vi "String to Boolean Array.vi"(8 "error in (no error)":errorcluster, 11 "String":string) -> (0 "error out":errorcluster, 2 "Array":bool[][](array[boolean]))   [LabVIEW 2026, in "LED Matrix.lvlib" / "Text.lvclass"]
uses:
  Text.lvclass
  Text.lvclass/Text.ctl
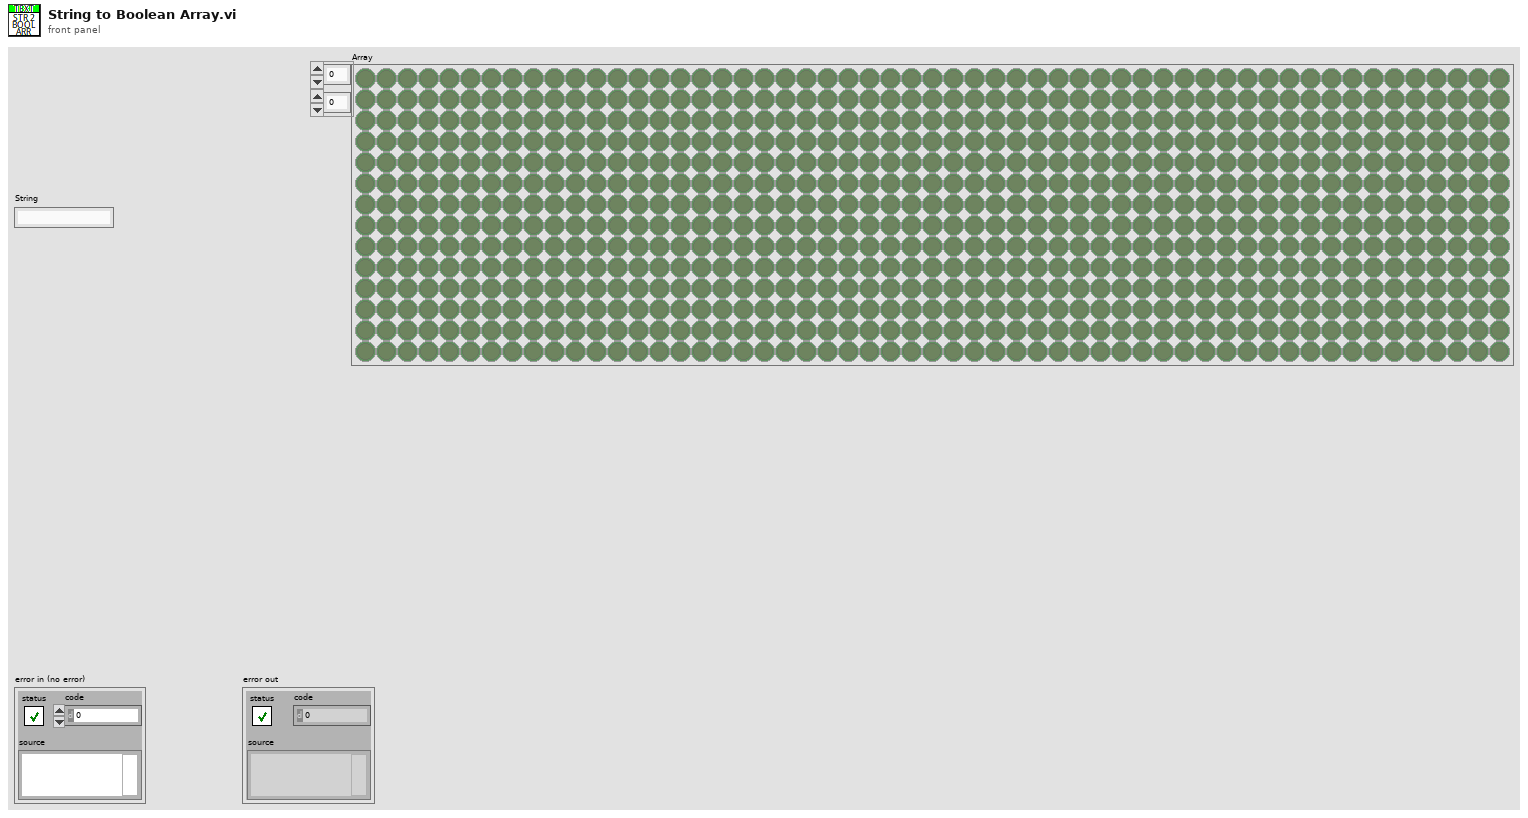
[diagram p1: front panel]
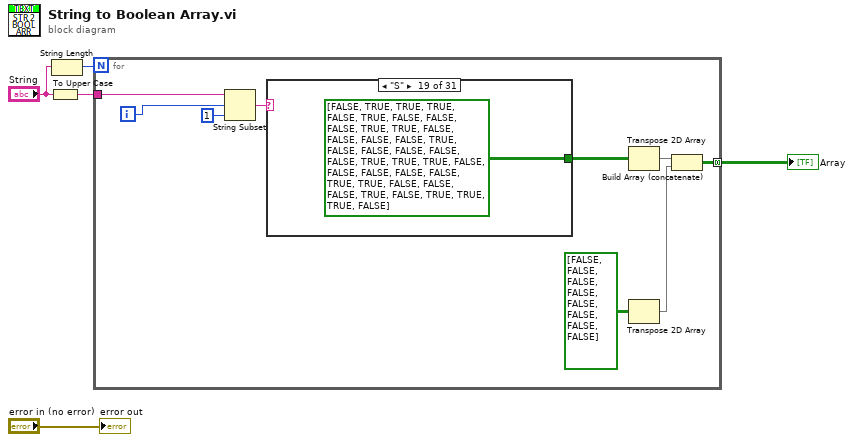
[diagram p0: block diagram]
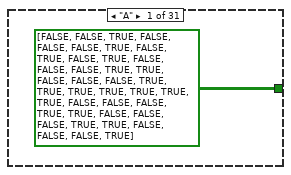
[diagram p2: hidden frame]
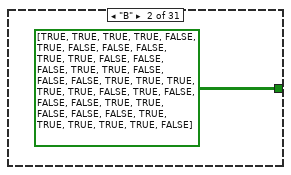
[diagram p3: hidden frame]
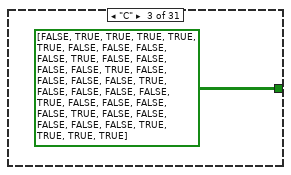
[diagram p4: hidden frame]
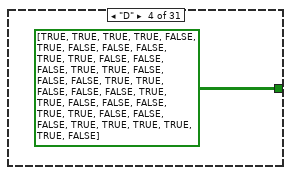
[diagram p5: hidden frame]
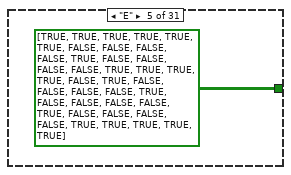
[diagram p6: hidden frame]
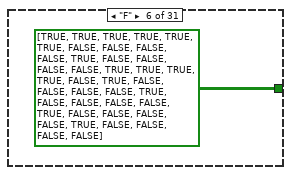
[diagram p7: hidden frame]
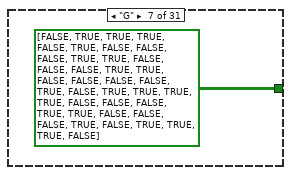
[diagram p8: hidden frame]
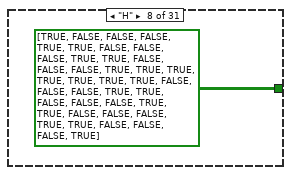
[diagram p9: hidden frame]
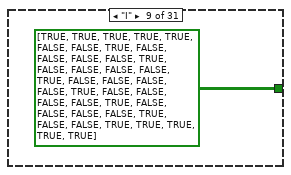
[diagram p10: hidden frame]
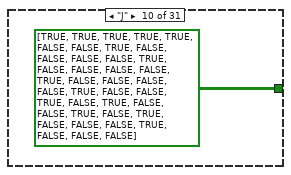
[diagram p11: hidden frame]
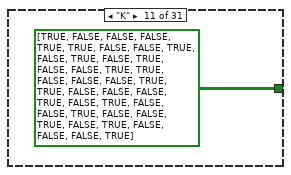
[diagram p12: hidden frame]
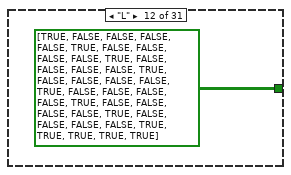
[diagram p13: hidden frame]
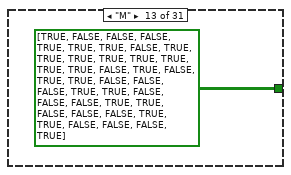
[diagram p14: hidden frame]
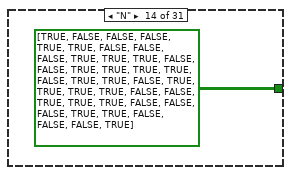
[diagram p15: hidden frame]
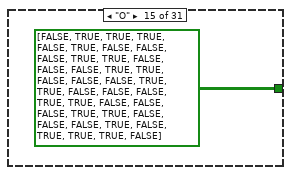
[diagram p16: hidden frame]
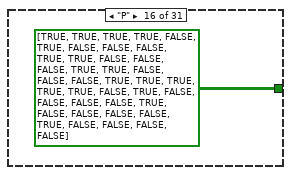
[diagram p17: hidden frame]
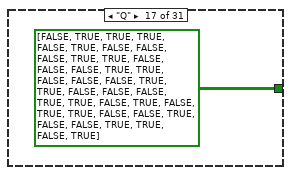
[diagram p18: hidden frame]
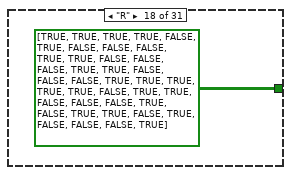
[diagram p19: hidden frame]
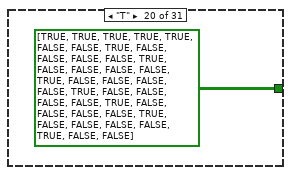
[diagram p20: hidden frame]
diagram:
  n1 = To Upper Case(1:"String") -> (0:w1:string)
  n2 = String Length(string="String") -> (length=w5:i32)
  n3 = for {
    N: w5 -> [_]
    tunnel: w1 -> [w14]
    tunnel: [w8] -> w3 mode=concatenating
    i -> [w9]
    n4 = String Subset(string=w14, offset (0)=w9, length (rest)=1 ("length (rest)")) -> (substring=w12:string)
    n5 = case shown="\"S\"" w12 {
      tunnel: [bool[][] [[FALSE, FALSE, TRUE, FALSE, FALSE], [FALSE, TRUE, FALSE, TRUE, FALSE], [TRUE, FALSE, FALSE, FALSE, TRUE], [TRUE, FALSE, FALSE, FALSE, TRUE], [TRUE, TRUE, TRUE, TRUE, TRUE], [TRUE, FALSE, FALSE, FALSE, TRUE], [TRUE, FALSE, FALSE, FALSE, TRUE], [TRUE, FALSE, FALSE, FALSE, TRUE]] bool[][] [[TRUE, TRUE, TRUE, TRUE, FALSE], [TRUE, FALSE, FALSE, FALSE, TRUE], [TRUE, FALSE, FALSE, FALSE, TRUE], [TRUE, FALSE, FALSE, FALSE, TRUE], [TRUE, TRUE, TRUE, TRUE, FALSE], [TRUE, FALSE, FALSE, FALSE, TRUE], [TRUE, FALSE, FALSE, FALSE, TRUE], [TRUE, TRUE, TRUE, TRUE, FALSE]] bool[][] [[FALSE, TRUE, TRUE, TRUE, TRUE], [TRUE, FALSE, FALSE, FALSE, FALSE], [TRUE, FALSE, FALSE, FALSE, FALSE], [TRUE, FALSE, FALSE, FALSE, FALSE], [TRUE, FALSE, FALSE, FALSE, FALSE], [TRUE, FALSE, FALSE, FALSE, FALSE], [TRUE, FALSE, FALSE, FALSE, FALSE], [FALSE, TRUE, TRUE, TRUE, TRUE]] bool[][] [[TRUE, TRUE, TRUE, TRUE, FALSE], [TRUE, FALSE, FALSE, FALSE, TRUE], [TRUE, FALSE, FALSE, FALSE, TRUE], [TRUE, FALSE, FALSE, FALSE, TRUE], [TRUE, FALSE, FALSE, FALSE, TRUE], [TRUE, FALSE, FALSE, FALSE, TRUE], [TRUE, FALSE, FALSE, FALSE, TRUE], [TRUE, TRUE, TRUE, TRUE, FALSE]] bool[][] [[TRUE, TRUE, TRUE, TRUE, TRUE], [TRUE, FALSE, FALSE, FALSE, FALSE], [TRUE, FALSE, FALSE, FALSE, FALSE], [TRUE, TRUE, TRUE, TRUE, FALSE], [TRUE, FALSE, FALSE, FALSE, FALSE], [TRUE, FALSE, FALSE, FALSE, FALSE], [TRUE, FALSE, FALSE, FALSE, FALSE], [TRUE, TRUE, TRUE, TRUE, TRUE]] bool[][] [[TRUE, TRUE, TRUE, TRUE, TRUE], [TRUE, FALSE, FALSE, FALSE, FALSE], [TRUE, FALSE, FALSE, FALSE, FALSE], [TRUE, TRUE, TRUE, TRUE, FALSE], [TRUE, FALSE, FALSE, FALSE, FALSE], [TRUE, FALSE, FALSE, FALSE, FALSE], [TRUE, FALSE, FALSE, FALSE, FALSE], [TRUE, FALSE, FALSE, FALSE, FALSE]] bool[][] [[FALSE, TRUE, TRUE, TRUE, FALSE], [TRUE, FALSE, FALSE, FALSE, TRUE], [TRUE, FALSE, FALSE, FALSE, TRUE], [TRUE, FALSE, FALSE, FALSE, FALSE], [TRUE, FALSE, TRUE, TRUE, TRUE], [TRUE, FALSE, FALSE, FALSE, TRUE], [TRUE, FALSE, FALSE, FALSE, TRUE], [FALSE, TRUE, TRUE, TRUE, FALSE]] bool[][] [[TRUE, FALSE, FALSE, FALSE, TRUE], [TRUE, FALSE, FALSE, FALSE, TRUE], [TRUE, FALSE, FALSE, FALSE, TRUE], [TRUE, TRUE, TRUE, TRUE, TRUE], [TRUE, FALSE, FALSE, FALSE, TRUE], [TRUE, FALSE, FALSE, FALSE, TRUE], [TRUE, FALSE, FALSE, FALSE, TRUE], [TRUE, FALSE, FALSE, FALSE, TRUE]] bool[][] [[TRUE, TRUE, TRUE, TRUE, TRUE], [FALSE, FALSE, TRUE, FALSE, FALSE], [FALSE, FALSE, TRUE, FALSE, FALSE], [FALSE, FALSE, TRUE, FALSE, FALSE], [FALSE, FALSE, TRUE, FALSE, FALSE], [FALSE, FALSE, TRUE, FALSE, FALSE], [FALSE, FALSE, TRUE, FALSE, FALSE], [TRUE, TRUE, TRUE, TRUE, TRUE]] bool[][] [[TRUE, TRUE, TRUE, TRUE, TRUE], [FALSE, FALSE, TRUE, FALSE, FALSE], [FALSE, FALSE, TRUE, FALSE, FALSE], [FALSE, FALSE, TRUE, FALSE, FALSE], [FALSE, FALSE, TRUE, FALSE, FALSE], [TRUE, FALSE, TRUE, FALSE, FALSE], [TRUE, FALSE, TRUE, FALSE, FALSE], [FALSE, TRUE, FALSE, FALSE, FALSE]] bool[][] [[TRUE, FALSE, FALSE, FALSE, TRUE], [TRUE, FALSE, FALSE, TRUE, FALSE], [TRUE, FALSE, TRUE, FALSE, FALSE], [TRUE, TRUE, FALSE, FALSE, FALSE], [TRUE, TRUE, FALSE, FALSE, FALSE], [TRUE, FALSE, TRUE, FALSE, FALSE], [TRUE, FALSE, FALSE, TRUE, FALSE], [TRUE, FALSE, FALSE, FALSE, TRUE]] bool[][] [[TRUE, FALSE, FALSE, FALSE, FALSE], [TRUE, FALSE, FALSE, FALSE, FALSE], [TRUE, FALSE, FALSE, FALSE, FALSE], [TRUE, FALSE, FALSE, FALSE, FALSE], [TRUE, FALSE, FALSE, FALSE, FALSE], [TRUE, FALSE, FALSE, FALSE, FALSE], [TRUE, FALSE, FALSE, FALSE, FALSE], [TRUE, TRUE, TRUE, TRUE, TRUE]] bool[][] [[TRUE, FALSE, FALSE, FALSE, TRUE], [TRUE, TRUE, FALSE, TRUE, TRUE], [TRUE, TRUE, TRUE, TRUE, TRUE], [TRUE, FALSE, TRUE, FALSE, TRUE], [TRUE, FALSE, FALSE, FALSE, TRUE], [TRUE, FALSE, FALSE, FALSE, TRUE], [TRUE, FALSE, FALSE, FALSE, TRUE], [TRUE, FALSE, FALSE, FALSE, TRUE]] bool[][] [[TRUE, FALSE, FALSE, FALSE, TRUE], [TRUE, FALSE, FALSE, FALSE, TRUE], [TRUE, TRUE, FALSE, FALSE, TRUE], [TRUE, TRUE, TRUE, FALSE, TRUE], [TRUE, FALSE, TRUE, TRUE, TRUE], [TRUE, FALSE, FALSE, TRUE, TRUE], [TRUE, FALSE, FALSE, FALSE, TRUE], [TRUE, FALSE, FALSE, FALSE, TRUE]] bool[][] [[FALSE, TRUE, TRUE, TRUE, FALSE], [TRUE, FALSE, FALSE, FALSE, TRUE], [TRUE, FALSE, FALSE, FALSE, TRUE], [TRUE, FALSE, FALSE, FALSE, TRUE], [TRUE, FALSE, FALSE, FALSE, TRUE], [TRUE, FALSE, FALSE, FALSE, TRUE], [TRUE, FALSE, FALSE, FALSE, TRUE], [FALSE, TRUE, TRUE, TRUE, FALSE]] bool[][] [[TRUE, TRUE, TRUE, TRUE, FALSE], [TRUE, FALSE, FALSE, FALSE, TRUE], [TRUE, FALSE, FALSE, FALSE, TRUE], [TRUE, FALSE, FALSE, FALSE, TRUE], [TRUE, TRUE, TRUE, TRUE, FALSE], [TRUE, FALSE, FALSE, FALSE, FALSE], [TRUE, FALSE, FALSE, FALSE, FALSE], [TRUE, FALSE, FALSE, FALSE, FALSE]] bool[][] [[FALSE, TRUE, TRUE, TRUE, FALSE], [TRUE, FALSE, FALSE, FALSE, TRUE], [TRUE, FALSE, FALSE, FALSE, TRUE], [TRUE, FALSE, FALSE, FALSE, TRUE], [TRUE, FALSE, FALSE, FALSE, TRUE], [TRUE, FALSE, TRUE, FALSE, TRUE], [TRUE, FALSE, FALSE, TRUE, FALSE], [FALSE, TRUE, TRUE, FALSE, TRUE]] bool[][] [[TRUE, TRUE, TRUE, TRUE, FALSE], [TRUE, FALSE, FALSE, FALSE, TRUE], [TRUE, FALSE, FALSE, FALSE, TRUE], [TRUE, FALSE, FALSE, FALSE, TRUE], [TRUE, TRUE, TRUE, TRUE, FALSE], [TRUE, TRUE, FALSE, FALSE, FALSE], [TRUE, FALSE, TRUE, TRUE, FALSE], [TRUE, FALSE, FALSE, FALSE, TRUE]] bool[][] [[FALSE, TRUE, TRUE, TRUE, FALSE], [TRUE, FALSE, FALSE, FALSE, TRUE], [TRUE, FALSE, FALSE, FALSE, FALSE], [TRUE, FALSE, FALSE, FALSE, FALSE], [FALSE, TRUE, TRUE, TRUE, FALSE], [FALSE, FALSE, FALSE, FALSE, TRUE], [TRUE, FALSE, FALSE, FALSE, TRUE], [FALSE, TRUE, TRUE, TRUE, FALSE]] bool[][] [[TRUE, TRUE, TRUE, TRUE, TRUE], [FALSE, FALSE, TRUE, FALSE, FALSE], [FALSE, FALSE, TRUE, FALSE, FALSE], [FALSE, FALSE, TRUE, FALSE, FALSE], [FALSE, FALSE, TRUE, FALSE, FALSE], [FALSE, FALSE, TRUE, FALSE, FALSE], [FALSE, FALSE, TRUE, FALSE, FALSE], [FALSE, FALSE, TRUE, FALSE, FALSE]] bool[][] [[TRUE, FALSE, FALSE, FALSE, TRUE], [TRUE, FALSE, FALSE, FALSE, TRUE], [TRUE, FALSE, FALSE, FALSE, TRUE], [TRUE, FALSE, FALSE, FALSE, TRUE], [TRUE, FALSE, FALSE, FALSE, TRUE], [TRUE, FALSE, FALSE, FALSE, TRUE], [TRUE, FALSE, FALSE, FALSE, TRUE], [FALSE, TRUE, TRUE, TRUE, FALSE]] bool[][] [[TRUE, FALSE, FALSE, FALSE, TRUE], [TRUE, FALSE, FALSE, FALSE, TRUE], [TRUE, FALSE, FALSE, FALSE, TRUE], [TRUE, FALSE, FALSE, FALSE, TRUE], [FALSE, TRUE, FALSE, TRUE, FALSE], [FALSE, TRUE, FALSE, TRUE, FALSE], [FALSE, TRUE, FALSE, TRUE, FALSE], [FALSE, FALSE, TRUE, FALSE, FALSE]] bool[][] [[TRUE, FALSE, FALSE, FALSE, FALSE, FALSE, FALSE, FALSE, TRUE], [TRUE, FALSE, FALSE, FALSE, FALSE, FALSE, FALSE, FALSE, TRUE], [TRUE, FALSE, FALSE, FALSE, FALSE, FALSE, FALSE, FALSE, TRUE], [TRUE, FALSE, FALSE, FALSE, TRUE, FALSE, FALSE, FALSE, TRUE], [FALSE, TRUE, FALSE, TRUE, FALSE, TRUE, FALSE, TRUE, FALSE], [FALSE, TRUE, FALSE, TRUE, FALSE, TRUE, FALSE, TRUE, FALSE], [FALSE, TRUE, FALSE, TRUE, FALSE, TRUE, FALSE, TRUE, FALSE], [FALSE, FALSE, TRUE, FALSE, FALSE, FALSE, TRUE, FALSE, FALSE]] bool[][] [[TRUE, FALSE, FALSE, FALSE, FALSE, FALSE, FALSE, TRUE], [FALSE, TRUE, FALSE, FALSE, FALSE, FALSE, TRUE, FALSE], [FALSE, FALSE, TRUE, FALSE, FALSE, TRUE, FALSE, FALSE], [FALSE, FALSE, FALSE, TRUE, TRUE, FALSE, FALSE, FALSE], [FALSE, FALSE, FALSE, TRUE, TRUE, FALSE, FALSE, FALSE], [FALSE, FALSE, TRUE, FALSE, FALSE, TRUE, FALSE, FALSE], [FALSE, TRUE, FALSE, FALSE, FALSE, FALSE, TRUE, FALSE], [TRUE, FALSE, FALSE, FALSE, FALSE, FALSE, FALSE, TRUE]] bool[][] [[TRUE, FALSE, FALSE, FALSE, FALSE, FALSE, TRUE], [FALSE, TRUE, FALSE, FALSE, FALSE, TRUE, FALSE], [FALSE, FALSE, TRUE, FALSE, TRUE, FALSE, FALSE], [FALSE, FALSE, FALSE, TRUE, FALSE, FALSE, FALSE], [FALSE, FALSE, FALSE, TRUE, FALSE, FALSE, FALSE], [FALSE, FALSE, FALSE, TRUE, FALSE, FALSE, FALSE], [FALSE, FALSE, FALSE, TRUE, FALSE, FALSE, FALSE], [FALSE, FALSE, FALSE, TRUE, FALSE, FALSE, FALSE]] bool[][] [[TRUE, TRUE, TRUE, TRUE, TRUE, TRUE, TRUE, TRUE], [FALSE, FALSE, FALSE, FALSE, FALSE, FALSE, TRUE, FALSE], [FALSE, FALSE, FALSE, FALSE, FALSE, TRUE, FALSE, FALSE], [FALSE, FALSE, FALSE, FALSE, TRUE, FALSE, FALSE, FALSE], [FALSE, FALSE, FALSE, TRUE, FALSE, FALSE, FALSE, FALSE], [FALSE, FALSE, TRUE, FALSE, FALSE, FALSE, FALSE, FALSE], [FALSE, TRUE, FALSE, FALSE, FALSE, FALSE, FALSE, FALSE], [TRUE, TRUE, TRUE, TRUE, TRUE, TRUE, TRUE, TRUE]] bool[][] [[TRUE], [TRUE], [TRUE], [TRUE], [TRUE], [TRUE], [TRUE], [TRUE]] bool[][] [[TRUE], [TRUE], [TRUE], [TRUE], [TRUE], [TRUE], [FALSE], [TRUE]] bool[][] [[FALSE, TRUE, TRUE, TRUE, FALSE, FALSE], [TRUE, FALSE, FALSE, FALSE, TRUE, FALSE], [TRUE, FALSE, FALSE, TRUE, FALSE, FALSE], [FALSE, TRUE, TRUE, FALSE, FALSE, FALSE], [FALSE, TRUE, TRUE, FALSE, FALSE, TRUE], [TRUE, FALSE, FALSE, TRUE, TRUE, FALSE], [TRUE, FALSE, FALSE, TRUE, TRUE, FALSE], [FALSE, TRUE, TRUE, FALSE, FALSE, TRUE]] bool[][] [[FALSE, FALSE, FALSE], [FALSE, FALSE, FALSE], [FALSE, FALSE, FALSE], [FALSE, FALSE, FALSE], [FALSE, FALSE, FALSE], [FALSE, FALSE, FALSE], [FALSE, FALSE, FALSE], [FALSE, FALSE, FALSE]] _] -> w11
      frame "A" {
      }
      frame "B" {
      }
      frame "C" {
      }
      frame "D" {
      }
      frame "E" {
      }
      frame "F" {
      }
      frame "G" {
      }
      frame "H" {
      }
      frame "I" {
      }
      frame "J" {
      }
      frame "K" {
      }
      frame "L" {
      }
      frame "M" {
      }
      frame "N" {
      }
      frame "O" {
      }
      frame "P" {
      }
      frame "Q" {
      }
      frame "R" {
      }
      frame "S" {
      }
      frame "T" {
      }
      frame "U" {
      }
      frame "V" {
      }
      frame "W" {
      }
      frame "X" {
      }
      frame "Y" {
      }
      frame "Z" {
      }
      frame "|" {
      }
      frame "!" {
      }
      frame "&" {
      }
      frame " " {
      }
      frame Default {
      }
    }
    n6 = Transpose 2D Array(2D array=w11) -> (transposed array=w7:bool[][])
    n7 = Transpose 2D Array(2D array=bool[][] [[FALSE], [FALSE], [FALSE], [FALSE], [FALSE], [FALSE], [FALSE], [FALSE]]) -> (transposed array=w6:bool[][])
    n8 = Build Array (concatenate)(w7, w6) -> (w8:bool[][])
  }
  "Array" <- w3
  "error out" <- "error in (no error)"
